vi "Load Hardware.vi"(8 "error in (no error)":errorcluster, 10 "Program only changes":bool=TRUE, 11 "Aerotech_Soloist in":refnum<class "Aerotech_Soloist.lvclass">) -> (0 "error out":errorcluster, 3 "Aerotech_Soloist out":refnum<class "Aerotech_Soloist.lvclass">)   [LabVIEW 2013, in "Aerotech_Soloist.lvclass"]
uses:
  Aerotech_Soloist.lvclass
  Device/Device.lvclass
panel:
  # "encapsulate HWI in cluser so each \"last encountered\"\ncan be a different length."
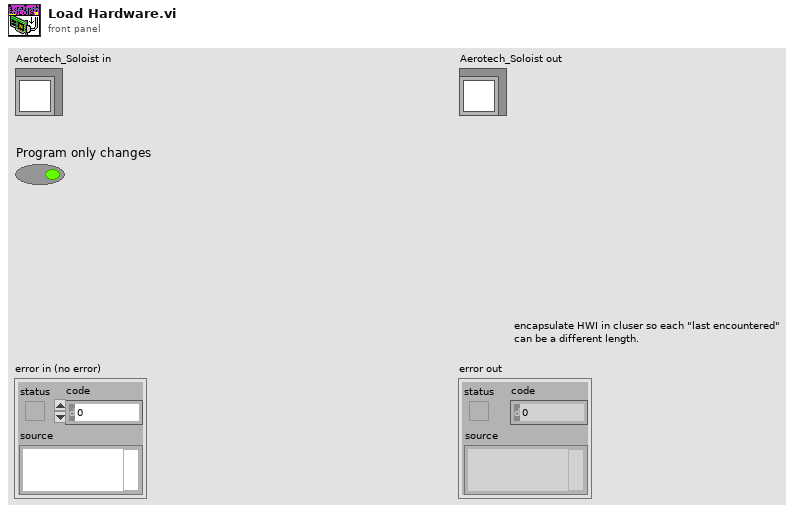
[diagram p1: front panel]
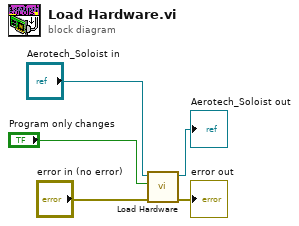
[diagram p0: block diagram]
diagram:
  n1 = call-parent "Load Hardware.vi"("error in (no error)"="error in (no error)", "Program only changes"="Program only changes", "Device in"="Aerotech_Soloist in") -> ("error out"=→"error out":errorcluster, "Device out"=→"Aerotech_Soloist out":refnum<class "Aerotech_Soloist.lvclass">)  [unwired: 7 in]
